vi "digital communication with buried intellengence.vi"() -> ()   [LabVIEW 2013]
uses:
  <vilib>/Analysis/3filter.llb/Filter Passband Type.ctl
  <vilib>/Analysis/3filter.llb/IIR Filter (DBL).vi
  <vilib>/Analysis/3filter.llb/Butterworth Filter (DBL).vi
  <vilib>/Analysis/3filter.llb/FIR Filter (DBL).vi
  <vilib>/Analysis/NI_AALBase.lvlib
panel:
  out "Numeric":u8
  out "hex integer string":string
  out "The original string hidden inside the image":string
  out "element":u32
  in  "file path (use dialog)":path
  out "image  with text file 2":picture
  out "image  with decoded data":picture
  out "image  with encoded data":picture
  out "Converted string":string
  in  "Desired Output Type":enum16{"Hexadecimal", "Binary"}(ring)
  in  "user choice of filter  blue channel":u16(ring) items=["Low-pass", "High-pass", "Band-pass", "Band-stop", "Bessel", "Elliptic"]
  in  "user choice of filter  green channel":u16(ring) items=["Low-pass", "High-pass", "Band-pass", "Band-stop", "Bessel", "Elliptic"]
  in  "user choice of noise 3 blue channel":u16(ring) items=["uniform white noise", "gaussian white noise", "periodic random noise", "no noise"]
  in  "user choice of noise 2 green channel":u16(ring) items=["uniform white noise", "gaussian white noise", "periodic random noise", "no noise"]
  out "image after filtration":picture
  out "image with noise":picture
  in  "user choice of filter red channel":u16(ring) items=["Low-pass", "High-pass", "Band-pass", "Band-stop", "Bessel", "Elliptic"]
  in  "user choice of noise, red channel":u16(ring) items=["uniform white noise", "gaussian white noise", "periodic random noise", "no noise"]
  out "input image":picture
  out "image":u8[](array[numeric])
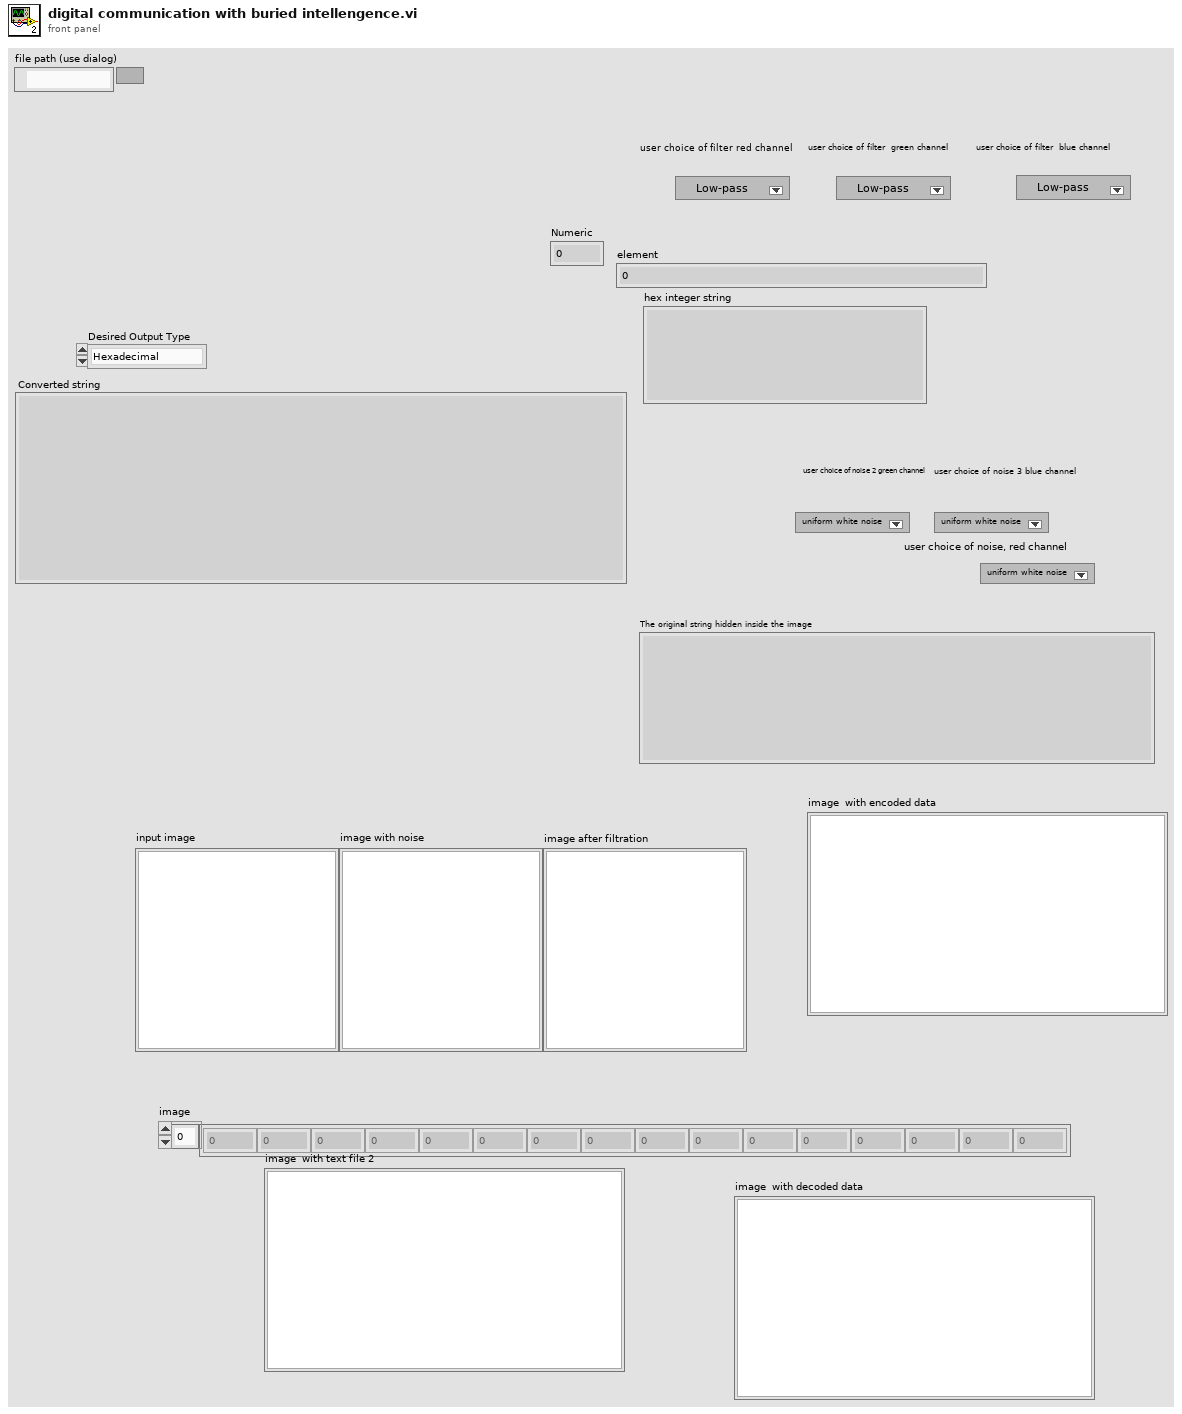
[diagram p1: front panel]
types:
  T1 = typedef "imagedata.ctl" = cluster{"image type":i32, "image depth":i32, "image":u8[], "mask":u8[], "colors":u32[], "Rectangle":cluster{"left":i16, "top":i16, "right":i16, "bottom":i16}}
  T2 = typedef "NI_AALBase.lvlib/Filter Passband Type.ctl" = enum32{"Lowpass", "Highpass", "Bandpass", "Bandstop"}
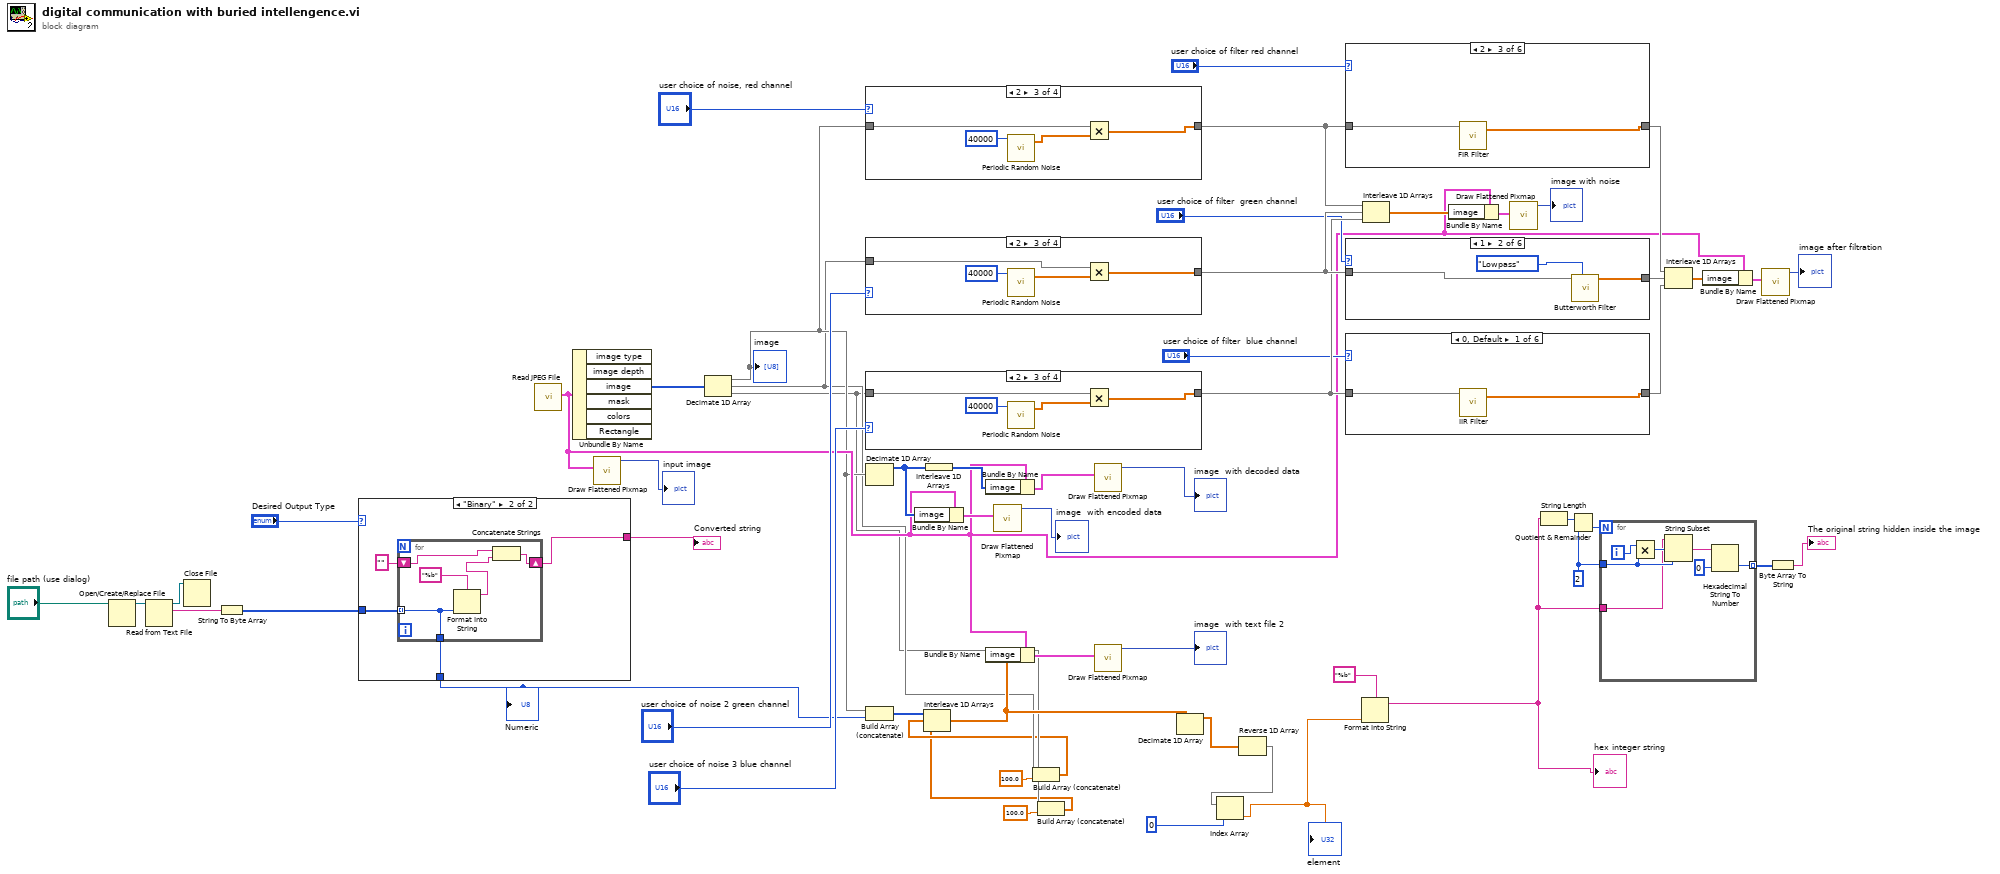
[diagram p0: block diagram]
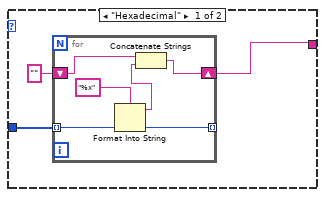
[diagram p2: hidden frame]
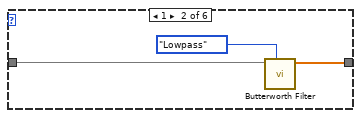
[diagram p3: hidden frame]
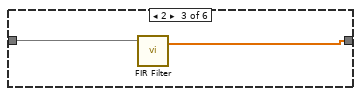
[diagram p4: hidden frame]
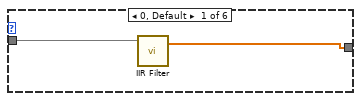
[diagram p8: hidden frame]
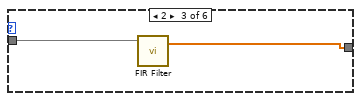
[diagram p9: hidden frame]
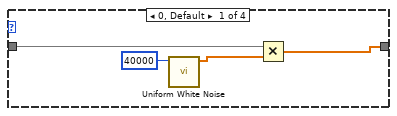
[diagram p13: hidden frame]
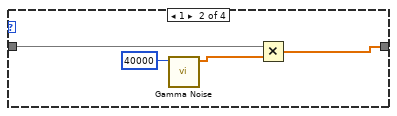
[diagram p14: hidden frame]
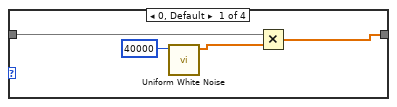
[diagram p16: hidden frame]
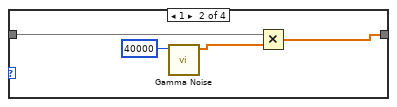
[diagram p17: hidden frame]
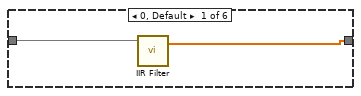
[diagram p19: hidden frame]
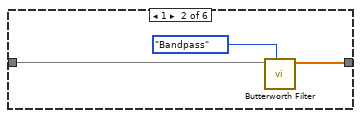
[diagram p20: hidden frame]
diagram:
  w8 = 2 ("y")
  n1 = Open/Create/Replace File(file path (use dialog)="file path (use dialog)") -> (refnum out=w37:refnum<file>)  [unwired: 5 in, 2 out]
  n2 = Read from Text File(file (use dialog)=w37) -> (refnum out=w38:refnum<file>, text=w36:string)  [unwired: 3 in, 2 out]
  n3 = Close File(refnum=w38) -> ()  [unwired: 1 in, 2 out]
  n4 = String To Byte Array(string=w36) -> (unsigned byte array=w39:u8[])
  n5 = case shown="\"Binary\"" "Desired Output Type" {
    tunnel: w39 -> [w60 w69]
    tunnel: [w58 w67] -> w6
    tunnel: [_ w66] -> w2
    frame "Hexadecimal" {
      n6 = for {
        tunnel: w60 -> [w61] mode=indexing
        shift-right: [w63] -> w58
        shift-left: "" -> [w64]
        tunnel: [w61] -> _ mode=indexing
        n7 = Format Into String(format string="%x", w61) -> (resulting string=w62:string)  [unwired: 2 in, 1 out]
        n8 = Concatenate Strings(w64, w62) -> (w63:string)
      }
    }
    frame "Binary" {
      n9 = for {
        shift-right: [w71] -> w67
        shift-left: "" -> [w73]
        tunnel: w69 -> [w70] mode=indexing
        tunnel: [w70] -> w66
        n10 = Format Into String(format string="%b", w70) -> (resulting string=w72:string)  [unwired: 2 in, 1 out]
        n11 = Concatenate Strings(w73, w72) -> (w71:string)
      }
    }
  }
  "Converted string" <- w6
  "Numeric" <- w2
  n12 = call <vilib>:"Read JPEG File.vi"() -> ("image data"=w26:T1)  [unwired: 9 in, 2 out]
  n13 = Unbundle By Name(w26) -> ("image"=w34:u8[])  [unwired: 5 out]
  n14 = call <vilib>:"Draw Flattened Pixmap.vi"("image data"=w26) -> ("new picture"=→"input image":picture)  [unwired: 8 in]
  n15 = Decimate 1D Array(w34) -> (w24:u8[], w15:u8[], w14:u8[])
  "image" <- w24
  n16 = case shown="2" "user choice of noise, red channel" {
    tunnel: w24 -> [w76 w81 w83 w87]
    tunnel: [w78 w80 w85 w87] -> w54
    frame 0, Default {
      n17 = call <vilib>:"Uniform White Noise.vi"("samples"=40000) -> ("uniform white noise"=w77:dbl[])  [unwired: 9 in, 1 out]
      n18 = Multiply(x=w76, y=w77) -> (x*y=w78:dbl[])
    }
    frame 1 {
      n19 = call <vilib>:"Gamma Noise.vi"("samples"=40000) -> ("gamma noise"=w82:dbl[])  [unwired: 9 in, 1 out]
      n20 = Multiply(x=w81, y=w82) -> (x*y=w80:dbl[])
    }
    frame 2 {
      n21 = call <vilib>:"Periodic Random Noise.vi"("samples"=40000) -> ("periodic random noise"=w86:dbl[])  [unwired: 2 in, 1 out]
      n22 = Multiply(x=w83, y=w86) -> (x*y=w85:dbl[])
    }
    frame 3 {
    }
  }
  n23 = case shown="2" "user choice of noise 2 green channel" {
    tunnel: [w90 w94 w99 w100] -> w52
    tunnel: w15 -> [w89 w93 w98 w100]
    frame 0, Default {
      n24 = call <vilib>:"Uniform White Noise.vi"("samples"=40000) -> ("uniform white noise"=w91:dbl[])  [unwired: 9 in, 1 out]
      n25 = Multiply(x=w89, y=w91) -> (x*y=w90:dbl[])
    }
    frame 1 {
      n26 = call <vilib>:"Gamma Noise.vi"("samples"=40000) -> ("gamma noise"=w95:dbl[])  [unwired: 9 in, 1 out]
      n27 = Multiply(x=w93, y=w95) -> (x*y=w94:dbl[])
    }
    frame 2 {
      n28 = call <vilib>:"Periodic Random Noise.vi"("samples"=40000) -> ("periodic random noise"=w97:dbl[])  [unwired: 2 in, 1 out]
      n29 = Multiply(x=w98, y=w97) -> (x*y=w99:dbl[])
    }
    frame 3 {
    }
  }
  n30 = case shown="2" "user choice of noise 3 blue channel" {
    tunnel: [w103 w107 w111 w113] -> w51
    tunnel: w14 -> [w102 w106 w110 w113]
    frame 0, Default {
      n31 = call <vilib>:"Uniform White Noise.vi"("samples"=40000) -> ("uniform white noise"=w104:dbl[])  [unwired: 9 in, 1 out]
      n32 = Multiply(x=w102, y=w104) -> (x*y=w103:dbl[])
    }
    frame 1 {
      n33 = call <vilib>:"Gamma Noise.vi"("samples"=40000) -> ("gamma noise"=w108:dbl[])  [unwired: 9 in, 1 out]
      n34 = Multiply(x=w106, y=w108) -> (x*y=w107:dbl[])
    }
    frame 2 {
      n35 = call <vilib>:"Periodic Random Noise.vi"("samples"=40000) -> ("periodic random noise"=w112:dbl[])  [unwired: 2 in, 1 out]
      n36 = Multiply(x=w110, y=w112) -> (x*y=w111:dbl[])
    }
    frame 3 {
    }
  }
  n37 = Decimate 1D Array(w24) -> (w30:u8[])  [unwired: 2 out]
  n38 = Build Array (concatenate)(w24, w2) -> (w3:u8[])
  n39 = Bundle By Name(cluster=w26, "image"=w30) -> (w32:T1)
  n40 = Interleave 1D Arrays(w30) -> (w29:u8[])
  n41 = Bundle By Name(cluster=w26, "image"=w29) -> (w28:T1)
  n42 = call <vilib>:"Draw Flattened Pixmap.vi"("image data"=w32) -> ("new picture"=→"image  with encoded data":picture)  [unwired: 8 in]
  n43 = Build Array (concatenate)(w15, 100.0 ("y")) -> (w13:dbl[])
  n44 = Build Array (concatenate)(w14, 100.0 ("y")) -> (w12:dbl[])
  n45 = Interleave 1D Arrays(w3, w13, w12) -> (w20:dbl[])
  n46 = Bundle By Name(cluster=w26, "image"=w20) -> (w23:T1)
  n47 = call <vilib>:"Draw Flattened Pixmap.vi"("image data"=w28) -> ("new picture"=→"image  with decoded data":picture)  [unwired: 8 in]
  n48 = call <vilib>:"Draw Flattened Pixmap.vi"("image data"=w23) -> ("new picture"=→"image  with text file 2":picture)  [unwired: 8 in]
  n49 = Decimate 1D Array(w20) -> (w19:dbl[])  [unwired: 2 out]
  n50 = Reverse 1D Array(array=w19) -> (reversed array=w18:dbl[])
  n51 = Index Array(array=w18, index=0) -> (element=w5:dbl)
  "element" <- w5
  n52 = case shown="2" "user choice of filter red channel" {
    tunnel: [w115 w118 w120 w121 w122 w123] -> w50
    tunnel: w54 -> [w114 w117 w119 w121 w122 w123]
    frame 0, Default {
      n53 = call-poly <vilib>:"IIR Filter.vi"("X"=w114) -> ("Filtered X"=w115:dbl[])  [unwired: 3 in, 1 out]
    }
    frame 1 {
      n54 = call-poly <vilib>:"Butterworth Filter.vi"("filter type"=Filter_Passband_Type."Bandpass", "X"=w117) -> ("Filtered X"=w118:dbl[])  [unwired: 6 in, 1 out]
    }
    frame 2 {
      n55 = call-poly <vilib>:"FIR Filter.vi"("X"=w119) -> ("Filtered X"=w120:dbl[])  [unwired: 3 in, 1 out]
    }
    frame 3 {
    }
    frame 4 {
    }
    frame 5 {
    }
  }
  n56 = case shown="1" "user choice of filter  green channel" {
    tunnel: [w125 w128 w130 w131 w132 w133] -> w49
    tunnel: w52 -> [w124 w127 w129 w131 w132 w133]
    frame 0, Default {
      n57 = call-poly <vilib>:"IIR Filter.vi"("X"=w124) -> ("Filtered X"=w125:dbl[])  [unwired: 3 in, 1 out]
    }
    frame 1 {
      n58 = call-poly <vilib>:"Butterworth Filter.vi"("filter type"=Filter_Passband_Type."Lowpass", "X"=w127) -> ("Filtered X"=w128:dbl[])  [unwired: 6 in, 1 out]
    }
    frame 2 {
      n59 = call-poly <vilib>:"FIR Filter.vi"("X"=w129) -> ("Filtered X"=w130:dbl[])  [unwired: 3 in, 1 out]
    }
    frame 3 {
    }
    frame 4 {
    }
    frame 5 {
    }
  }
  n60 = case shown="0, Default" "user choice of filter  blue channel" {
    tunnel: [w135 w138 w140 w141 w142 w143] -> w48
    tunnel: w51 -> [w134 w137 w139 w141 w142 w143]
    frame 0, Default {
      n61 = call-poly <vilib>:"IIR Filter.vi"("X"=w134) -> ("Filtered X"=w135:dbl[])  [unwired: 3 in, 1 out]
    }
    frame 1 {
      n62 = call-poly <vilib>:"Butterworth Filter.vi"("filter type"=Filter_Passband_Type."Lowpass", "X"=w137) -> ("Filtered X"=w138:dbl[])  [unwired: 6 in, 1 out]
    }
    frame 2 {
      n63 = call-poly <vilib>:"FIR Filter.vi"("X"=w139) -> ("Filtered X"=w140:dbl[])  [unwired: 3 in, 1 out]
    }
    frame 3 {
    }
    frame 4 {
    }
    frame 5 {
    }
  }
  n64 = Format Into String(format string="%b", w5) -> (resulting string=w4:string)  [unwired: 2 in, 1 out]
  "hex integer string" <- w4
  n65 = Interleave 1D Arrays(w54, w52, w51) -> (w46:dbl[])
  n66 = Bundle By Name(cluster=w26, "image"=w46) -> (w57:T1)
  n67 = call <vilib>:"Draw Flattened Pixmap.vi"("image data"=w57) -> ("new picture"=→"image with noise":picture)  [unwired: 8 in]
  n68 = String Length(string=w4) -> (length=w10:i32)
  n69 = Quotient & Remainder(x=w10, y=w8) -> (floor(x/y)=w9:i32)  [unwired: 1 out]
  n70 = for {
    N: w9 -> [_]
    tunnel: [w149] -> w11 mode=indexing
    tunnel: w8 -> [w145]
    tunnel: w4 -> [w144]
    i -> [w146]
    n71 = Multiply(x=w146, y=w145) -> (x*y=w147:i32)
    n72 = String Subset(string=w144, offset (0)=w147, length (rest)=w145) -> (substring=w148:string)
    n73 = Hexadecimal String To Number(string=w148, default (0uL)=u8 0) -> (number=w149:u8)  [unwired: 1 in, 1 out]
  }
  n74 = Interleave 1D Arrays(w50, w49, w48) -> (w45:dbl[])
  n75 = Bundle By Name(cluster=w26, "image"=w45) -> (w55:T1)
  n76 = call <vilib>:"Draw Flattened Pixmap.vi"("image data"=w55) -> ("new picture"=→"image after filtration":picture)  [unwired: 8 in]
  n77 = Byte Array To String(unsigned byte array=w11) -> (string=→"The original string hidden inside the image":string)
